vi "name.vi"(6 "sample name":string="cance4r", 7 "Save directory":path=path "\\\\157.82.9.50\\d/HW/b11 cance4r", 9 "tempro number":i32, 10 "batch#":string, 11 "laser channel":string) -> (1 "temprory data name":string, 2 "time stamp":string, 3 "file naming":string)   [LabVIEW 2021]
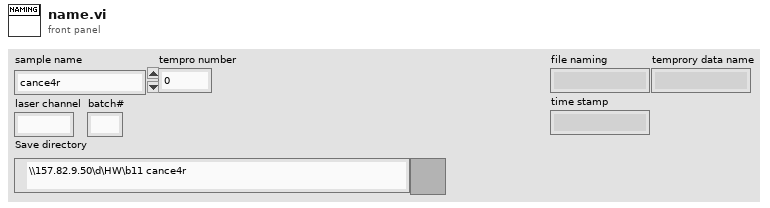
[diagram p1: front panel]
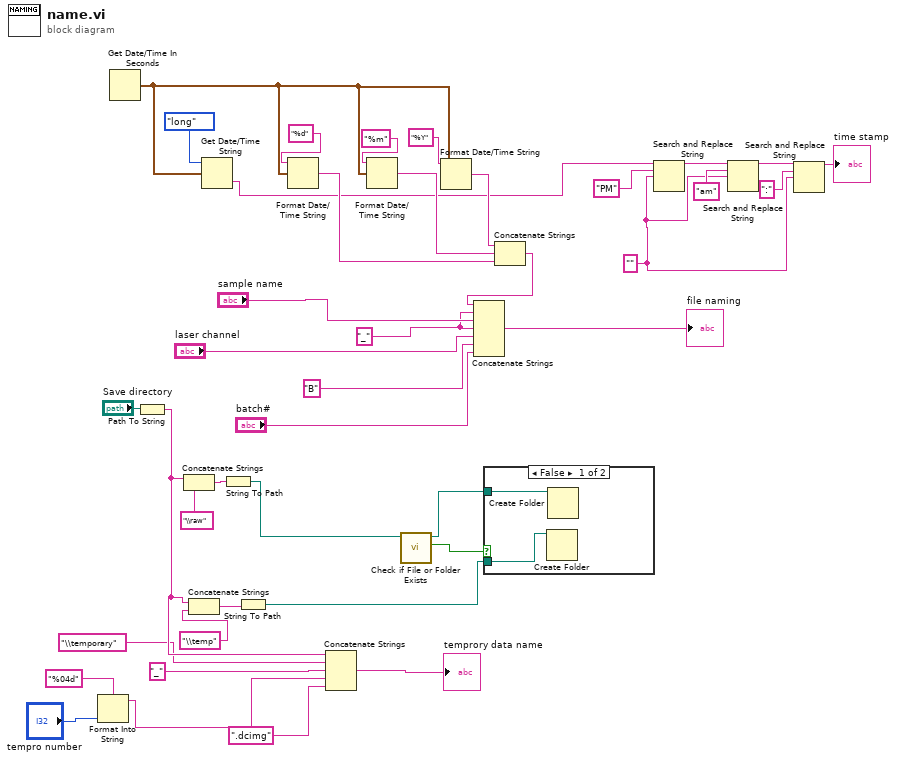
[diagram p0: block diagram]
diagram:
  w9 = "" ("replace string (\"\")")
  w22 = "_" ("string")
  n1 = Format Into String(format string="%04d" ("initial string"), "tempro number") -> (resulting string=w6:string)  [unwired: 2 in, 1 out]
  n2 = Get Date/Time In Seconds() -> (seconds since 1Jan1904=w28:timestamp)
  n3 = Path To String(path="Save directory") -> (string=w3:string)
  n4 = Concatenate Strings(w3, "\\raw") -> (w38:string)
  n5 = Concatenate Strings(w3, "\\temp") -> (w35:string)
  n6 = Get Date/Time String(date format (0)=enum16{"short", "long", "abbreviated"}."long", seconds (now)=w28) -> (time string=w15:string)  [unwired: 1 in, 1 out]
  n7 = String To Path(string=w38) -> (path=w37:path)
  n8 = String To Path(string=w35) -> (path=w34:path)
  n9 = Format Date/Time String(time format string (%c)="%d", seconds (now)=w28) -> (date/time string=w25:string)  [unwired: 1 in]
  n10 = Concatenate Strings(w3, "\\temporary" ("initial string"), "_" ("string"), w6, ".dcimg" ("string")) -> (→"temprory data name":string)
  n11 = Format Date/Time String(time format string (%c)="%m", seconds (now)=w28) -> (date/time string=w26:string)  [unwired: 1 in]
  n12 = call <vilib>:"Check if File or Folder Exists.vi"("path"=w37) -> ("file or folder exists?"=w39:bool, "dup path"=w33:path)  [unwired: 8 in, 1 out]
  n13 = Format Date/Time String(time format string (%c)="%Y", seconds (now)=w28) -> (date/time string=w27:string)  [unwired: 1 in]
  n14 = case shown="False" w39 {
    tunnel: w34 -> [w42 _]
    tunnel: w33 -> [w41 _]
    frame False {
      n15 = Create Folder(path (use dialog)=w42) -> ()  [unwired: 2 in, 3 out]
      n16 = Create Folder(path (use dialog)=w41) -> ()  [unwired: 2 in, 3 out]
    }
    frame True {
    }
  }
  n17 = Concatenate Strings(w27, w26, w25) -> (w24:string)
  n18 = Concatenate Strings(w24, w22, "sample name", w22, "laser channel", "B" ("string"), "batch#") -> (→"file naming":string)
  n19 = Search and Replace String(input string=w15, search string="PM", replace string=w9) -> (result string=w14:string)  [unwired: 5 in, 3 out]
  n20 = Search and Replace String(input string=w14, search string="am", replace string=w9) -> (result string=w12:string)  [unwired: 5 in, 3 out]
  n21 = Search and Replace String(input string=w12, search string=":", replace string=w9) -> (result string=→"time stamp":string)  [unwired: 5 in, 3 out]
